vi "Shoot_Hot_Command.vi"(10 "Delay ms":u32=500) -> ()   [LabVIEW 2014]
uses:
  TORC Code/GlobalVariable.vi
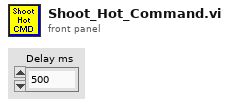
[diagram p1: front panel]
types:
  T1 = enum16{"Unready", "Ready", "Clear", "Fire", "Reload", "Arm In"}
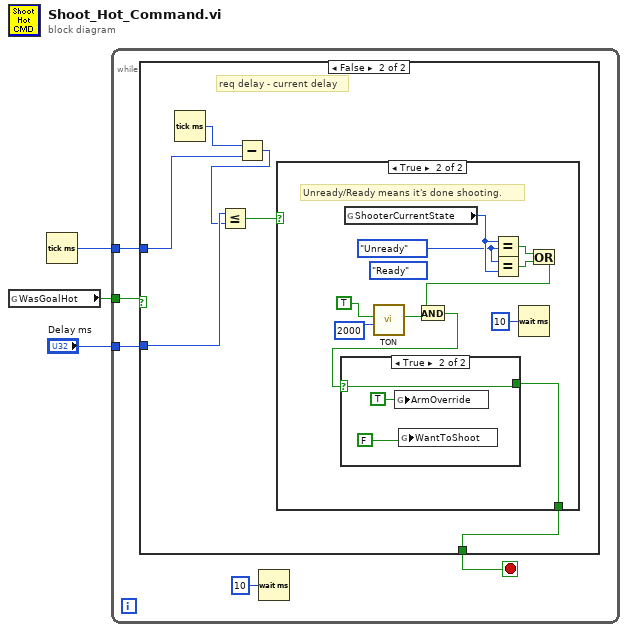
[diagram p0: block diagram]
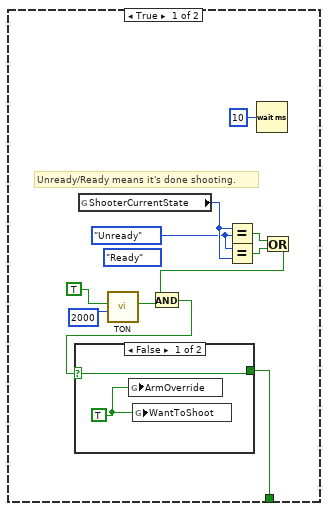
[diagram p2: hidden frame]
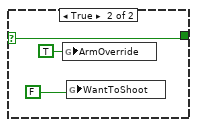
[diagram p3: hidden frame]
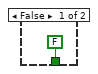
[diagram p4: hidden frame]
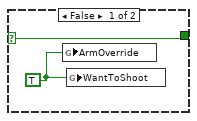
[diagram p5: hidden frame]
diagram:
  n1 = global read "GlobalVariable.vi" "WasGoalHot"() -> (w3:bool)
  n2 = Tick Count (ms)() -> (millisecond timer value=w1:u32)
  n3 = while {
    tunnel: w3 -> [w8]
    tunnel: "Delay ms" -> [w7]
    tunnel: w1 -> [w5]
    stop <- w6 stop-if-true
    n4 = case shown="False" w8 {
      tunnel: w7 -> [_ w27]
      tunnel: [w9 w30] -> w6
      tunnel: w5 -> [_ w28]
      frame True {
        (unwired) T1."Ready" ("y")
        w16 = T1."Unready" ("y")
        # "Unready/Ready means it's done shooting."
        n5 = global read "GlobalVariable.vi" "ShooterCurrentState"() -> (w17:T1)
        n6 = call "TON.vi"("Delay (ms)"=u32 2000 ("Delay ms"), "Input"=TRUE ("WantToShoot")) -> ("Output"=w14:bool)  [unwired: 9 in]
        n7 = Equal?(x=w17, y=w16) -> (x = y?=w18:bool)
        n8 = Equal?(x=w16, y=w17) -> (x = y?=w15:bool)
        n9 = Wait (ms)(milliseconds to wait=u32 10) -> ()  [unwired: 1 out]
        n10 = Or(x=w18, y=w15) -> (x .or. y?=w13:bool)
        n11 = And(x=w13, y=w14) -> (x .and. y?=w11:bool)
        n12 = case shown="False" w11 {
          selector: w11 -> [w20 w23]
          tunnel: [w20 w23] -> w9
          frame False {
            w21 = TRUE ("WantToShoot")
            n13 = global write "GlobalVariable.vi" "ArmOverride"(w21) -> ()
            n14 = global write "GlobalVariable.vi" "WantToShoot"(w21) -> ()
          }
          frame True {
            n15 = global write "GlobalVariable.vi" "ArmOverride"(TRUE ("ArmOverride")) -> ()
            n16 = global write "GlobalVariable.vi" "WantToShoot"(FALSE ("WantToShoot")) -> ()
          }
        }
      }
      frame False {
        # "req delay - current delay"
        n17 = Tick Count (ms)() -> (millisecond timer value=w29:u32)
        n18 = Subtract(x=w29, y=w28) -> (x-y=w26:u32)
        n19 = Less Or Equal?(x=w27, y=w26) -> (x <= y?=w25:bool)
        n20 = case shown="True" w25 {
          tunnel: [FALSE w32] -> w30
          frame False {
          }
          frame True {
            (unwired) T1."Ready" ("y")
            w39 = T1."Unready" ("y")
            # "Unready/Ready means it's done shooting."
            n21 = global read "GlobalVariable.vi" "ShooterCurrentState"() -> (w40:T1)
            n22 = call "TON.vi"("Delay (ms)"=u32 2000 ("Delay ms"), "Input"=TRUE ("WantToShoot")) -> ("Output"=w37:bool)  [unwired: 9 in]
            n23 = Equal?(x=w40, y=w39) -> (x = y?=w41:bool)
            n24 = Equal?(x=w39, y=w40) -> (x = y?=w38:bool)
            n25 = Wait (ms)(milliseconds to wait=u32 10) -> ()  [unwired: 1 out]
            n26 = Or(x=w41, y=w38) -> (x .or. y?=w36:bool)
            n27 = And(x=w36, y=w37) -> (x .and. y?=w33:bool)
            n28 = case shown="True" w33 {
              selector: w33 -> [w43 w46]
              tunnel: [w43 w46] -> w32
              frame False {
                w44 = TRUE ("WantToShoot")
                n29 = global write "GlobalVariable.vi" "ArmOverride"(w44) -> ()
                n30 = global write "GlobalVariable.vi" "WantToShoot"(w44) -> ()
              }
              frame True {
                n31 = global write "GlobalVariable.vi" "ArmOverride"(TRUE ("ArmOverride")) -> ()
                n32 = global write "GlobalVariable.vi" "WantToShoot"(FALSE ("WantToShoot")) -> ()
              }
            }
          }
        }
      }
    }
    n33 = Wait (ms)(milliseconds to wait=u32 10 ("millisecond multiple")) -> ()  [unwired: 1 out]
  }
